vi "Set_Parameter_Instrument (Json).vi"(8 "error in (no error)":errorcluster caption="entrée d'erreur (pas d'erreur)", 10 "Parameter (Json)":string, 11 "Show_Information en entrée":refnum<class "Wait_Voltage.lvclass">) -> (0 "error out":errorcluster caption="sortie d'erreur", 3 "Show_Information en sortie":refnum<class "Wait_Voltage.lvclass">)   [LabVIEW 2020, in "Library Test.lvlib" / "Wait_Voltage.lvclass"]
uses:
  Wait_Voltage.lvclass
  C:/Users/ngarcin/OneDrive - Altyor/Standard TB/Class/Test/Test (Default)/Test (Default).lvclass
  Wait_Voltage.lvclass/Wait_Voltage.ctl
  JSON API/JSON Value/Set from JSON string.vi
  Test_Without_Instr/Test_Without_Inst.lvclass
  Instrument/Instrument (Default)/Class Instrument (Default).lvclass
  JSON API/JSON Value/JSON Value.lvclass
  JSON API/Variant JSON/Variant JSON.lvlib
  JSON API/Get Polymorphic/JSON GetSet.lvlib
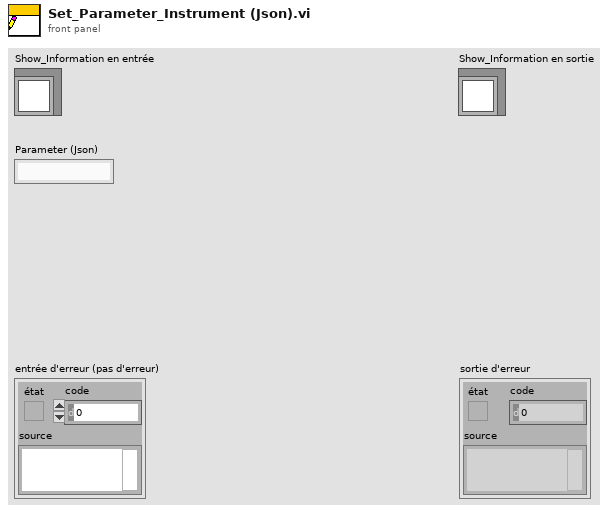
[diagram p1: front panel]
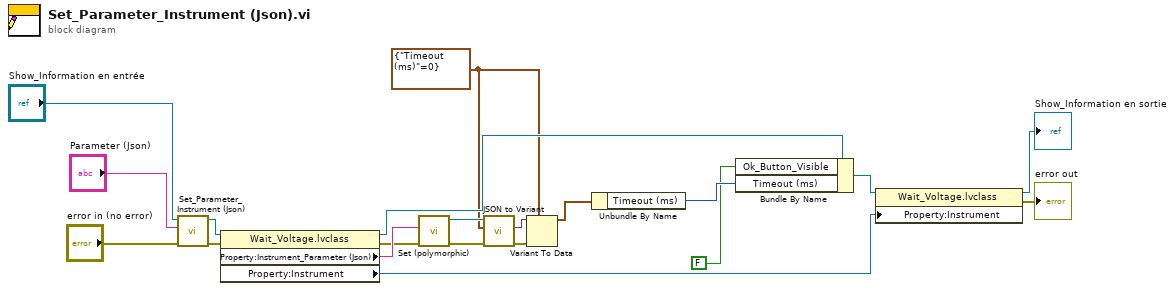
[diagram p0: block diagram]
diagram:
  w6 = cluster{"Timeout (ms)":u64} {"Timeout (ms)"=0} ("Cluster des données privées de classe")
  n1 = call-parent "Set_Parameter_Instrument (Json).vi"("error in (no error)"="error in (no error)", "Parameter (Json)"="Parameter (Json)", "Test (Default) en entrée"="Show_Information en entrée") -> ("error out"=w10:errorcluster, "Test (Default) en sortie"=w11:refnum<class "Wait_Voltage.lvclass">)  [unwired: 7 in]
  n2 = property class="Wait_Voltage.lvclass"(reference=w11, error in=w10) -> (reference out=w9:refnum<class "Wait_Voltage.lvclass">, error out=w16:errorcluster, "Property:Instrument_Parameter (Json)"=w17:string, "Property:Instrument"=w1:refnum<class "Class Instrument (Default).lvclass">)
  n3 = call-poly "Set (polymorphic).vi"("error in (no error)"=w16, "JSON stream"=w17) -> ("error out"=w13:errorcluster, "JSON Value out"=w15:refnum<class "JSON Value.lvclass">)  [unwired: 7 in, 1 out]
  n4 = call "JSON to Variant.vi"("error in (no error)"=w13, "Variant (Data Type)"=w6, "JSON Value"=w15) -> ("error out"=w14:errorcluster, "Variant out"=w12:variant)  [unwired: 7 in]
  n5 = Variant To Data(error in=w14, type=w6, Variant=w12) -> (data=w8:cluster{"Timeout (ms)":u64})  [unwired: 1 out]
  n6 = Unbundle By Name(w8) -> ("Timeout (ms)"=w7:u64)
  n7 = Bundle By Name(cluster=w9, "Ok_Button_Visible"=FALSE, "Timeout (ms)"=w7) -> (w5:refnum<class "Wait_Voltage.lvclass">)
  n8 = property class="Wait_Voltage.lvclass"(reference=w5, "Property:Instrument"=w1) -> (reference out=→"Show_Information en sortie":refnum<class "Wait_Voltage.lvclass">, error out=→"error out":errorcluster)  [unwired: 1 in]
